vi "GEM_BANK_Clear.vi"(8 "error in (no error)":errorcluster, 11 "LVBANK in":refnum<class "GEM_BANK.lvclass">) -> (0 "error out":errorcluster, 3 "LVBANK out":refnum<class "GEM_BANK.lvclass">)   [LabVIEW 2018, in "GEM_BANK.lvclass"]
uses:
  GEM_BANK.lvclass
  GEM_BANK.lvclass/GEM_BANK.ctl
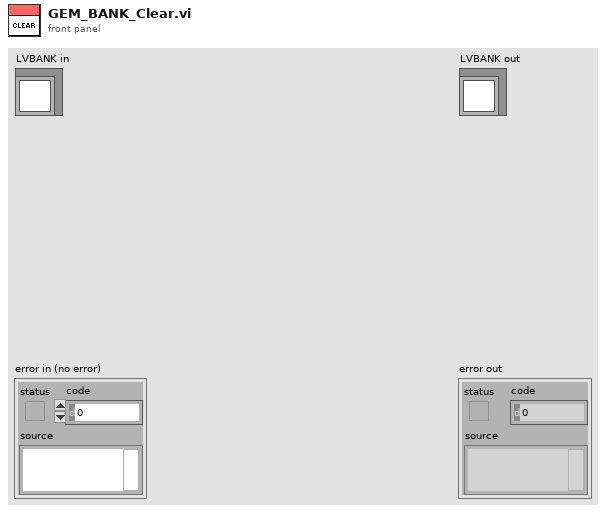
[diagram p1: front panel]
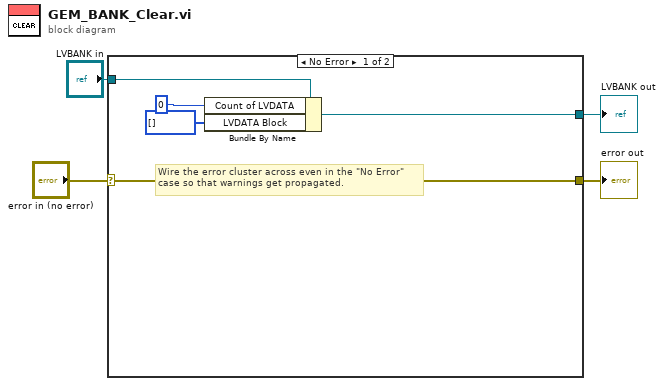
[diagram p0: block diagram]
diagram:
  n1 = case shown="No Error" "error in (no error)" {
    selector: "error in (no error)" -> [w9 w11]
    tunnel: [w9 w11] -> w3
    tunnel: [w8 w10] -> w1
    tunnel: "LVBANK in" -> [w6 w10]
    frame No Error {
      # "Wire the error cluster across even in the \"No Error\"\ncase so that warnings get propagated."
      n2 = Bundle By Name(cluster=w6, "Count of LVDATA"=0, "LVDATA Block"=u8[] []) -> (w8:refnum<class "GEM_BANK.lvclass">)
    }
    frame Error {
    }
  }
  "error out" <- w3
  "LVBANK out" <- w1
